vi "sub vi vi.vi"() -> ()   [LabVIEW 2012]
panel:
  out "cout":bool
  out "sum":bool
  in  "b":bool
  in  "a":bool
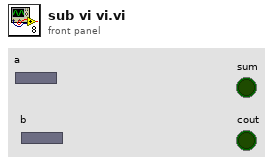
[diagram p1: front panel]
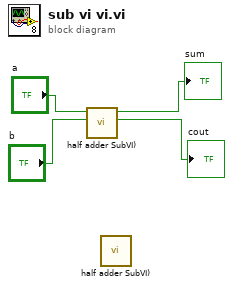
[diagram p0: block diagram]
diagram:
  n1 = call "half adder SubVI).vi"("b"="b", "a"="a") -> ("cout"=→"cout":bool, "sum"=→"sum":bool)  [unwired: 8 in]
  n2 = call "half adder SubVI).vi"() -> ()  [unwired: 2 in, 2 out]
